vi "XorRem.vi"(10 "Numeric 2":dbl, 11 "Numeric":dbl) -> (3 "Boolean":bool)   [LabVIEW 2014]
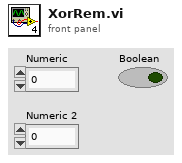
[diagram p1: front panel]
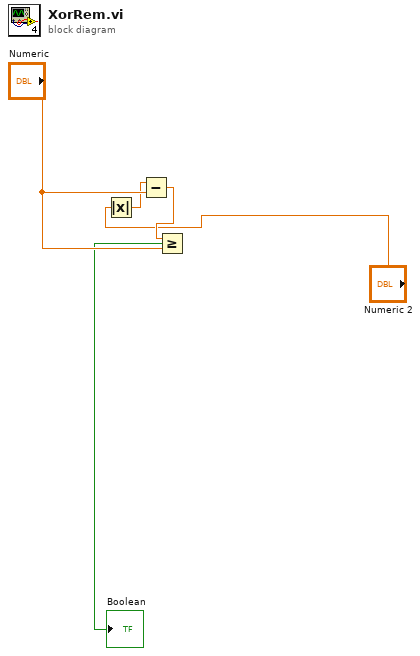
[diagram p0: block diagram]
diagram:
  n1 = Absolute Value(x="Numeric 2") -> (abs(x)=w3:dbl)
  n2 = Subtract(x=w3, y="Numeric") -> (x-y=w4:dbl)
  n3 = Greater Or Equal?(x=w4, y="Numeric") -> (x >= y?=→"Boolean":bool)
